vi "多影像平均_二值化.vi"() -> ()   [LabVIEW 2015]
uses:
  <vilib>/userdefined/High Color/IMAQdx.ctl
  <vilib>/vision/NI_Vision_Development_Module.lvlib
  <vilib>/vision/driver/NI_Vision_Acquisition_Software.lvlib
  <resource>/objmgr/imaqdx.rc
panel:
  out "error out":errorcluster
  out "影像陣列":T1[](array[plugin-control])
  out "Mean":sgl format="%#.2f"
  out "Standard Deviation":sgl format="%#.2f"
  out "平均影像Histograph":T2(graph)
  out "Image binary":T1(plugin-control)
  in  "stop":bool
  out "全部影像Histograph":T3(graph)
  in  "Horizontal Progress Bar":u8(slide) scale=0.0..255.0
  out "二值化影像陣列":T1[](array[plugin-control])
  out "取像視窗":T1(plugin-control)
  in  "Session In":T4="cam1"
  in  "載入影像":bool
  in  "拍攝影像":bool
  in  "影像數量":i32=4
  out "Image mean":T1(plugin-control)
  out "取像編號":i32
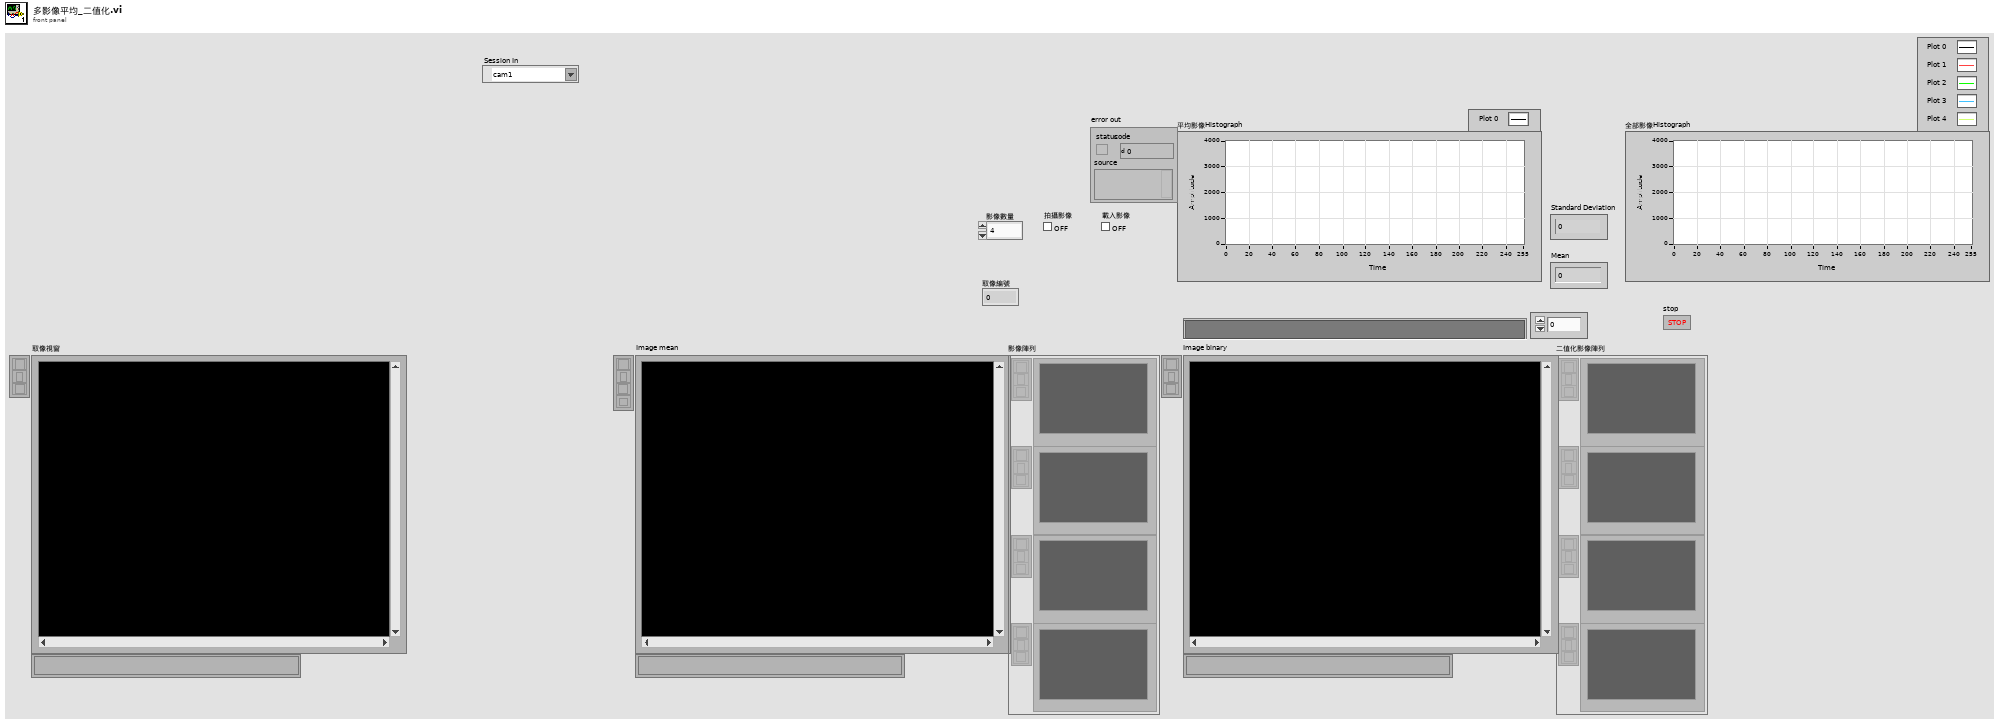
[diagram p1: front panel]
types:
  T1 = typedef "IMAQ Image.ctl" = refnum<image>
  T2 = cluster{"Starting Value":sgl, "Incremental Value":sgl, "Histogram":u32[]}
  T3 = cluster{"Starting Value":sgl, "Incremental Value":sgl, "Histogram":u32[]}[]
  T4 = typedef "IMAQdx.ctl" = refnum<k21>
  T5 = cluster{"Global Rectangle":i32[], "Contours":cluster{"Contour Type":u32, "ROI Type":u32, "Points":i32[]}[]}
  T6 = typedef "Image Type" = u32
  T7 = typedef "IMAQ Rectangle" = cluster{"Left":i32, "Top":i32, "Right":i32, "Bottom":i32, "Rotation":dbl}
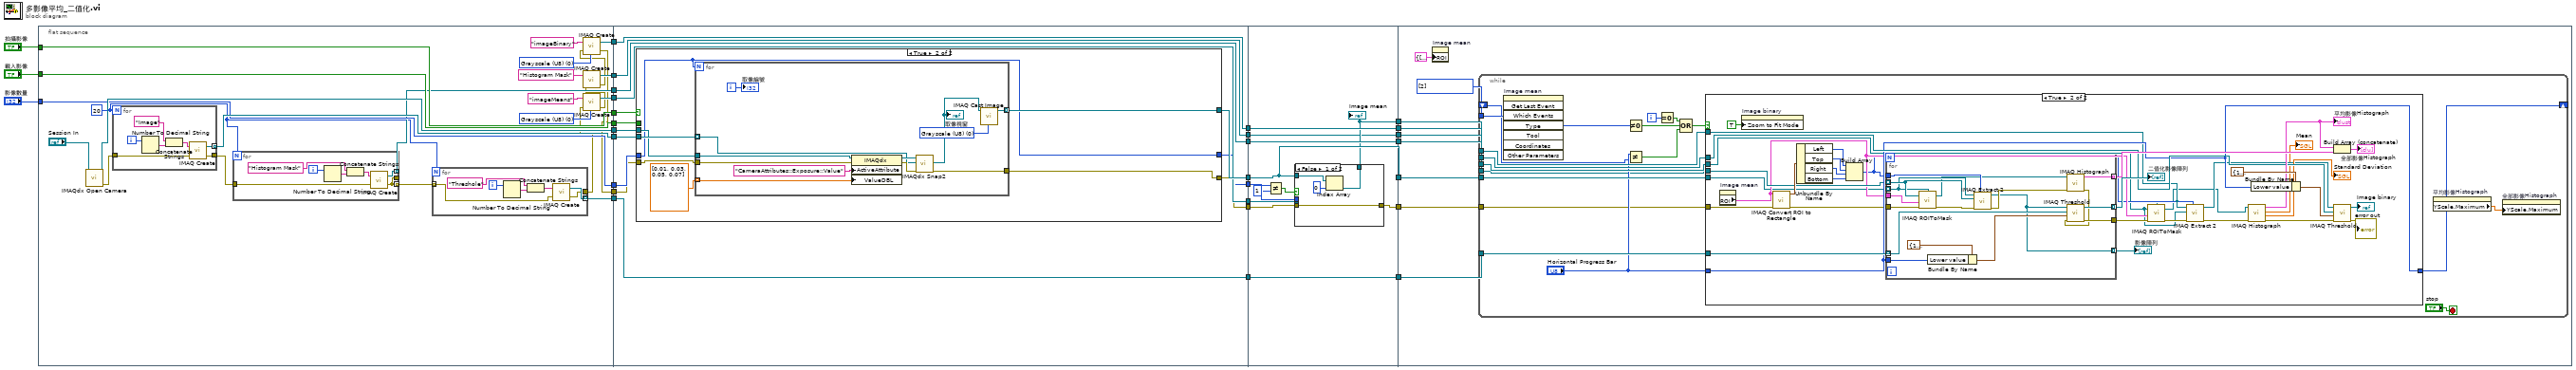
[diagram p0: block diagram]
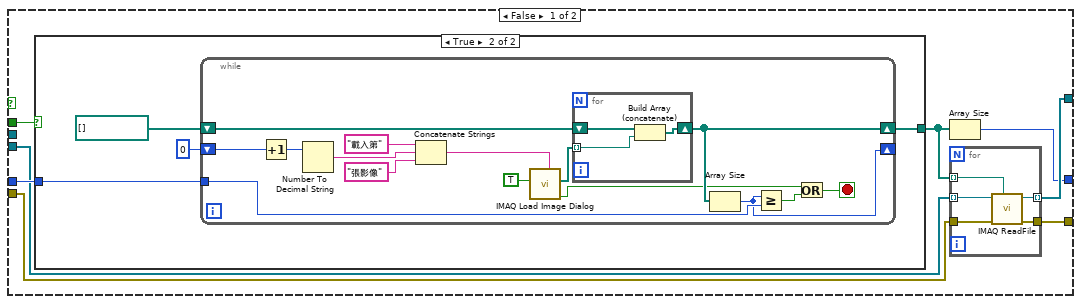
[diagram p2: hidden frame]
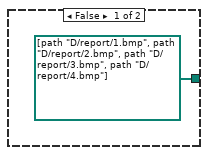
[diagram p3: hidden frame]
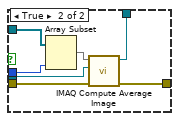
[diagram p4: hidden frame]
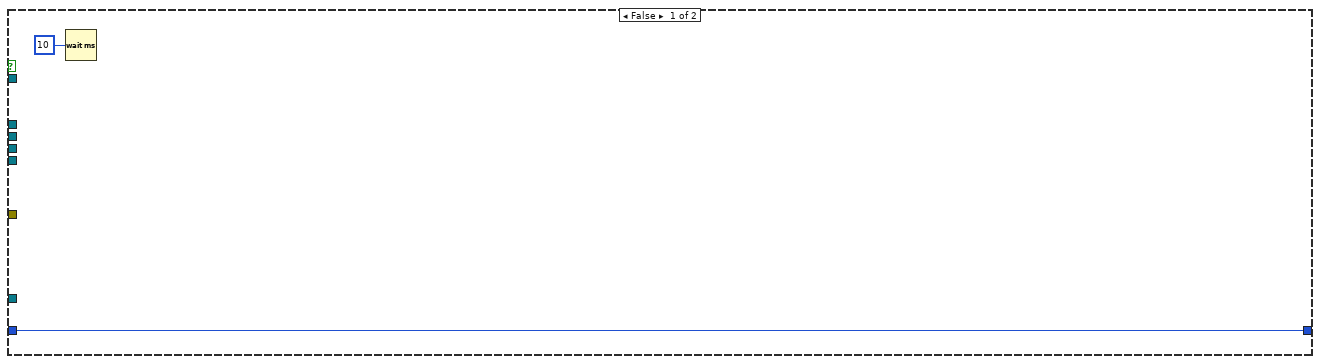
[diagram p5: hidden frame]
diagram:
  n1 = flat-sequence {
    tunnel: [w52] -> w29
    tunnel: [w51] -> w28
    tunnel: [w49] -> w26
    tunnel: "影像數量" -> [w45]
    tunnel: [w47] -> w23
    tunnel: "拍攝影像" -> [w47]
    tunnel: [w46] -> w21
    tunnel: "載入影像" -> [w46]
    tunnel: [w45] -> w19
    tunnel: [w44] -> w16
    tunnel: [w41] -> w8
    tunnel: [w39] -> w7
    tunnel: [w37] -> w2
    tunnel: [w30] -> w1
    tunnel: w29 -> [w87]
    tunnel: w28 -> [w88]
    tunnel: [w86] -> w27
    tunnel: w26 -> [w85]
    tunnel: [w85] -> w25
    tunnel: w23 -> [w84]
    tunnel: w21 -> [w83]
    tunnel: w19 -> [w82]
    tunnel: [w81] -> w18
    tunnel: [w80] -> w17
    tunnel: w16 -> [w79]
    tunnel: [w79] -> w15
    tunnel: [w78] -> w9
    tunnel: w8 -> [w78]
    tunnel: w7 -> [w77]
    tunnel: [w77] -> w6
    tunnel: [w76] -> w3
    tunnel: w2 -> [w76]
    tunnel: w1 -> [w75]
    tunnel: w27 -> [w149]
    tunnel: w25 -> [w155]
    tunnel: w18 -> [w154]
    tunnel: w17 -> [w146]
    tunnel: w15 -> [w153]
    tunnel: [w153] -> w14
    tunnel: [w150] -> w13
    tunnel: [w149] -> w12
    tunnel: [w148] -> w11
    tunnel: [w152] -> w10
    tunnel: w9 -> [w152]
    tunnel: w6 -> [w147]
    tunnel: [w147] -> w5
    tunnel: [w151] -> w4
    tunnel: w3 -> [w151]
    tunnel: w14 -> [w174]
    tunnel: w13 -> [w168]
    tunnel: w12 -> [w175]
    tunnel: w11 -> [w173]
    tunnel: w10 -> [w172]
    tunnel: w5 -> [w167]
    tunnel: w4 -> [w169]
    frame #0 {
      w43 = T6 0 items=["Grayscale (U8)", "Grayscale (I16)", "Grayscale (SGL)", "Complex (CSG)", "RGB (U32)", "HSL (U32)", "RGB (U64)", "Grayscale (U16)"] ("Image Type")
      w36 = 20
      w48 = T6 0 items=["Grayscale (U8)", "Grayscale (I16)", "Grayscale (SGL)", "Complex (CSG)", "RGB (U32)", "HSL (U32)", "RGB (U64)", "Grayscale (U16)"] ("Image Type")
      n2 = call <vilib>:"IMAQdx Open Camera.vi"("Session In"="Session In") -> ("error out"=w38:errorcluster, "Session Out"=w52:T4)  [unwired: 9 in]
      n3 = for {
        N: w36 -> [_]
        tunnel: [w74] -> w51 mode=indexing
        tunnel: w38 -> [w73]
        tunnel: [w72] -> w35
        i -> [w71]
        n4 = Number To Decimal String(number=w71) -> (decimal integer string=w69:string)  [unwired: 1 in]
        n5 = Concatenate Strings("Image", w69) -> (w68:string)
        n6 = call "IMAQ Create"("Image Name"=w68, "error in (no error)"=w73) -> ("New Image"=w74:T1, "error out"=w72:errorcluster)  [unwired: 3 in]
      }
      n7 = for {
        N: w36 -> [_]
        tunnel: [w60] -> w37 mode=indexing
        tunnel: w35 -> [w59]
        tunnel: [w54] -> _
        tunnel: [w54] -> w34 mode=indexing
        i -> [w58]
        n8 = Number To Decimal String(number=w58) -> (decimal integer string=w56:string)  [unwired: 1 in]
        n9 = Concatenate Strings("Histogram Mask", w56) -> (w55:string)
        n10 = call "IMAQ Create"("Image Name"=w55, "error in (no error)"=w59) -> ("New Image"=w60:T1, "error out"=w54:errorcluster)  [unwired: 3 in]
      }
      n11 = for {
        N: w36 -> [_]
        tunnel: [w67] -> w44 mode=indexing
        tunnel: w34 -> [w66] mode=indexing
        tunnel: [w65] -> w31
        i -> [w64]
        n12 = Number To Decimal String(number=w64) -> (decimal integer string=w62:string)  [unwired: 1 in]
        n13 = Concatenate Strings("Threshole", w62) -> (w61:string)
        n14 = call "IMAQ Create"("Image Name"=w61, "error in (no error)"=w66) -> ("New Image"=w67:T1, "error out"=w65:errorcluster)  [unwired: 3 in]
      }
      n15 = call "IMAQ Create"("Image Name"="imageMeans", "Image Type"=w48, "error in (no error)"=w31) -> ("New Image"=w49:T1, "error out"=w33:errorcluster)  [unwired: 2 in]
      n16 = call "IMAQ Create"("Image Name"="Histogram Mask", "error in (no error)"=w33) -> ("New Image"=w39:T1, "error out"=w32:errorcluster)  [unwired: 3 in]
      n17 = call "IMAQ Create"("Image Name"="imageBinary", "Image Type"=w43, "error in (no error)"=w32) -> ("New Image"=w41:T1, "error out"=w30:errorcluster)  [unwired: 2 in]
    }
    frame #1 {
      n18 = case shown="True" w84 {
        tunnel: w88 -> [w93 w131]
        tunnel: w87 -> [_ w130]
        tunnel: w75 -> [w92 w128]
        tunnel: [w94 w127] -> w86
        tunnel: w83 -> [w96 _]
        tunnel: w82 -> [w95 w125]
        tunnel: [w91 w126] -> w81
        tunnel: [w89 w125] -> w80
        frame False {
          n19 = case shown="True" w96 {
            tunnel: [path[] [path "D:/report/1.bmp", path "D:/report/2.bmp", path "D:/report/3.bmp", path "D:/report/4.bmp"] w101] -> w90
            tunnel: w95 -> [_ w100]
            frame False {
            }
            frame True {
              n20 = while {
                tunnel: w100 -> [w113]
                shift-right: [w116] -> w101
                shift-left: path[] [] -> [w112]
                shift-right: [w111] -> _
                shift-left: 0 -> [w110]
                stop <- w103 stop-if-true
                n21 = Increment(x=w110) -> (x+1=w109:i32)
                n22 = Number To Decimal String(number=w109) -> (decimal integer string=w106:string)  [unwired: 1 in]
                n23 = Concatenate Strings("載入第", w106, "張影像") -> (w105:string)
                n24 = call "IMAQ Load Image Dialog"("Button Label"=w105, "Multiple Files? (No)"=TRUE) -> ("Cancelled?"=w104:bool, "Paths"=w114:path[])  [unwired: 7 in, 1 out]
                n25 = for {
                  tunnel: w114 -> [w118] mode=indexing
                  shift-right: [w117] -> w116
                  shift-left: w112 -> [w119]
                  n26 = Build Array (concatenate)(w119, w118) -> (w117:path[])
                }
                n27 = Array Size(array=w116) -> (size(s)=w111:i32)
                n28 = Greater Or Equal?(x=w111, y=w113) -> (x >= y?=w102:bool)
                n29 = Or(x=w104, y=w102) -> (x .or. y?=w103:bool)
              }
            }
          }
          n30 = Array Size(array=w90) -> (size(s)=w89:i32)
          n31 = for {
            tunnel: w90 -> [w124] mode=indexing
            tunnel: [w123] -> w94 mode=indexing
            tunnel: w93 -> [w122] mode=indexing
            tunnel: w92 -> [w121]
            tunnel: [w120] -> w91
            n32 = call "IMAQ ReadFile"("File Path"=w124, "error in (no error)"=w121, "Image"=w122) -> ("error out"=w120:errorcluster, "Image Out"=w123:T1)  [unwired: 4 in, 3 out]
          }
        }
        frame True {
          n33 = for {
            N: w125 -> [_]
            tunnel: w131 -> [w132] mode=indexing
            tunnel: w130 -> [w142]
            tunnel: dbl[] [0.01, 0.03, 0.05, 0.07] -> [w141] mode=indexing
            tunnel: w128 -> [w136]
            tunnel: [w140] -> w127 mode=indexing
            tunnel: [w138] -> w126
            i -> [w143]
            w139 = T6 0 items=["Grayscale (U8)", "Grayscale (I16)", "Grayscale (SGL)", "Complex (CSG)", "RGB (U32)", "HSL (U32)", "RGB (U64)", "Grayscale (U16)"] ("Image Type")
            n34 = property class="IMAQdx"(reference=w142, error in=w136, "ActiveAttribute"="CameraAttributes::Exposure::Value", "ValueDBL"=w141) -> (reference out=w133:T4, error out=w135:errorcluster)
            n35 = call <vilib>:"IMAQdx Snap2.vi"("error in"=w135, "Image In"=w132, "Session In"=w133) -> ("error out"=w138:errorcluster, "Image Out"=w137:T1)  [unwired: 6 in, 1 out]
            "取像視窗" <- w137
            n36 = call "IMAQ Cast Image"("Image Type"=w139, "Image Src"=w137) -> ("Image Dst Out"=w140:T1)  [unwired: 8 in, 1 out]
            "取像編號" <- w143
          }
        }
      }
    }
    frame #2 {
      n37 = Not Equal?(x=w146, y=1) -> (x != y?=w144:bool)
      n38 = case shown="False" w144 {
        tunnel: w155 -> [_ w166]
        tunnel: w154 -> [w159 w165]
        tunnel: w146 -> [_ w164]
        tunnel: [w159 w162] -> w150
        tunnel: w149 -> [w157 w161]
        tunnel: [w156 w160] -> w148
        frame False {
          n39 = Index Array(array=w157, index=0) -> (element=w156:T1)
        }
        frame True {
          n40 = Array Subset(array=w161, length=w164) -> (w163:T1[])  [unwired: 1 in]
          n41 = call "IMAQ Compute Average Image"("error in (no error)"=w165, "Image Dst"=w166, "Images"=w163) -> ("error out"=w162:errorcluster, "Image Dst Out"=w160:T1)  [unwired: 7 in]
        }
      }
      "Image mean" <- w148
    }
    frame #3 {
      w170 = i32[] [2] items=["No  event", "Click event", "Draw event", "Move event", "Size event", "Scroll event", "Activate event", "Close event", "Double click event"] ("Events list (all)")
      n42 = property on="Image mean" class="ImageControl"("ROI"=T5 {"Global Rectangle"=[0, 0, 1292, 964], "Contours"=[{"Contour Type"=0, "ROI Type"=3, "Points"=[0, 0, 1292, 964]}]}) -> ()  [unwired: 2 in, 2 out]
      n43 = while {
        tunnel: w175 -> [w194]
        tunnel: w174 -> [w193]
        tunnel: w173 -> [w191]
        tunnel: w167 -> [w192]
        tunnel: w172 -> [w190]
        tunnel: w170 -> [w188]
        shift-right: [w185] -> _
        shift-left: _ -> [w183]
        tunnel: w169 -> [w178]
        tunnel: w168 -> [w177]
        i -> [w186]
        stop <- "stop" stop-if-true
        n44 = invoke on="Image mean" class="ImageControl" method="Get Last Event"("Which Events"=w188) -> ("Type"=w187:i32)  [unwired: 7 in, 7 out]
        n45 = Not Equal To 0?(x=w187) -> (x != 0?=w181:bool)
        n46 = Not Equal?(x="Horizontal Progress Bar", y=w183) -> (x != y?=w180:bool)
        n47 = Equal To 0?(x=w186) -> (x = 0?=w182:bool)
        n48 = Compound Arithmetic op=OR(w182, w181, w180) -> (w179:bool)
        n49 = case shown="True" w179 {
          tunnel: w194 -> [_ w202]
          tunnel: w193 -> [_ w230]
          tunnel: w192 -> [_ w199]
          tunnel: w191 -> [_ w200]
          tunnel: w190 -> [_ w217]
          tunnel: "Horizontal Progress Bar" -> [w195 w215]
          tunnel: [w195 w215] -> w185
          tunnel: w178 -> [_ w213]
          tunnel: w177 -> [_ w204]
          frame False {
            n50 = Wait (ms)(milliseconds to wait=u32 10) -> ()  [unwired: 1 out]
          }
          frame True {
            n51 = property on="Image mean" class="ImageControl"() -> ("ROI"=w212:T5)  [unwired: 2 in, 2 out]
            n52 = property on="Image binary" class="ImageControl"("Zoom to Fit Mode"=TRUE) -> ()  [unwired: 2 in, 2 out]
            n53 = call "IMAQ Convert ROI to Rectangle"("error in (no error)"=w204, "ROI Descriptor"=w212) -> ("error out"=w205:errorcluster, "Rectangle"=w222:T7)  [unwired: 7 in]
            n54 = Unbundle By Name(w222) -> ("Left"=w218:i32, "Top"=w219:i32, "Right"=w220:i32, "Bottom"=w221:i32)
            n55 = Build Array(w218, w219, w220, w221) -> (w211:i32[])
            n56 = for {
              tunnel: w202 -> [w233] mode=indexing
              tunnel: w230 -> [w247] mode=indexing
              tunnel: [w246] -> w229 mode=indexing
              tunnel: [w234] -> w225 mode=indexing
              tunnel: w215 -> [w243]
              tunnel: w213 -> [w240] mode=indexing
              tunnel: w212 -> [w242]
              tunnel: w211 -> [w241]
              tunnel: [w237] -> w206
              tunnel: w205 -> [w236]
              tunnel: [w235] -> w201 mode=indexing
              n57 = call "IMAQ ROIToMask"("error in (no error)"=w236, "ROI Descriptor"=w242, "Image"=w240, "Image Model"=w233) -> ("error out"=w239:errorcluster, "Image Out"=w232:T1)  [unwired: 2 in, 1 out]
              n58 = Bundle By Name(cluster=cluster{"Lower value":sgl, "Upper value":sgl} {"Lower value"=128.0, "Upper value"=255.0} ("Range"), "Lower value"=w243) -> (w244:cluster{"Lower value":sgl, "Upper value":sgl})
              n59 = call "IMAQ Extract 2"("Optional Rectangle"=w241, "error in (no error)"=w239, "Image Dst"=w240, "Image Src"=w233) -> ("error out"=w238:errorcluster, "Image Dst Out"=w235:T1)  [unwired: 6 in]
              n60 = call "IMAQ Histograph"("error in (no error)"=w238, "Image"=w232) -> ("error out"=w231:errorcluster, "Histogram Graph"=w234:T2)  [unwired: 6 in, 2 out]
              n61 = call "IMAQ Threshold"("error in (no error)"=w231, "Range"=w244, "Image Dst"=w247, "Image Src"=w235) -> ("error out"=w237:errorcluster, "Image Dst Out"=w246:T1)  [unwired: 6 in]
            }
            "二值化影像陣列" <- w229
            "影像陣列" <- w201
            n62 = call "IMAQ ROIToMask"("error in (no error)"=w206, "ROI Descriptor"=w212, "Image"=w199, "Image Model"=w200) -> ("error out"=w209:errorcluster, "Image Out"=w198:T1)  [unwired: 2 in, 1 out]
            n63 = call "IMAQ Extract 2"("Optional Rectangle"=w211, "error in (no error)"=w209, "Image Dst"=w199, "Image Src"=w200) -> ("error out"=w208:errorcluster, "Image Dst Out"=w210:T1)  [unwired: 6 in]
            n64 = call "IMAQ Histograph"("error in (no error)"=w208, "Image"=w198) -> ("error out"=w207:errorcluster, "Standard  Deviation"=→"Standard Deviation":sgl, "Mean Value"=→"Mean":sgl, "Histogram Graph"=w223:T2)  [unwired: 6 in]
            "平均影像Histograph" <- w223
            n65 = Bundle By Name(cluster=cluster{"Lower value":sgl, "Upper value":sgl} {"Lower value"=128.0, "Upper value"=255.0} ("Range"), "Lower value"=w215) -> (w228:cluster{"Lower value":sgl, "Upper value":sgl})
            n66 = Build Array (concatenate)(w223, w225) -> (→"全部影像Histograph":T3)
            n67 = call "IMAQ Threshold"("error in (no error)"=w207, "Range"=w228, "Image Dst"=w217, "Image Src"=w210) -> ("error out"=→"error out":errorcluster, "Image Dst Out"=→"Image binary":T1)  [unwired: 6 in]
          }
        }
        n68 = property on="平均影像Histograph" class="WFGraph (strict)"() -> ("YScale.Maximum"=w176:dbl)  [unwired: 2 in, 2 out]
        n69 = property on="全部影像Histograph" class="WFGraph (strict)"("YScale.Maximum"=w176) -> ()  [unwired: 2 in, 2 out]
      }
    }
  }
